vi "登录界面.vi"() -> ()   [LabVIEW 2023]
panel:
  in  "登录":bool
  in  "密   码":string
  in  "用户名":string
  # "登陆界面"
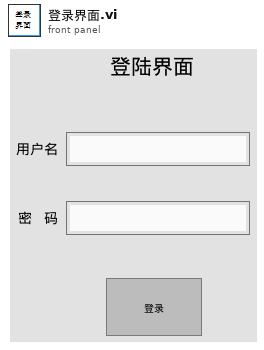
[diagram p1: front panel]
types:
  T1 = enum32{"Invalid", "Standard", "Closed", "Hidden", "Minimized", "Maximized"}
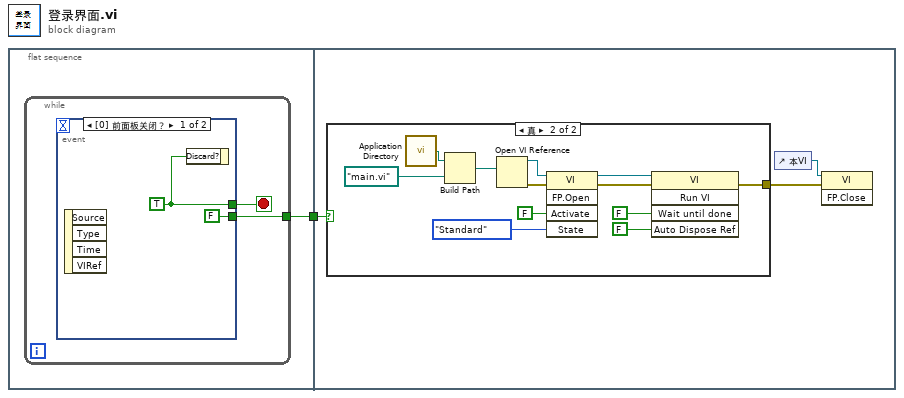
[diagram p0: block diagram]
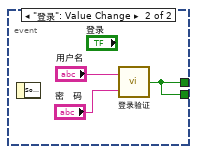
[diagram p2: hidden frame]
diagram:
  n1 = flat-sequence {
    tunnel: [w2] -> w1
    tunnel: w1 -> [w10]
    frame #0 {
      n2 = while {
        tunnel: [w3] -> w2
        stop <- w4 stop-if-true
        n3 = event shown="[0] 前面板关闭？" {
          selector: _ -> [_ _]
          dyn-events: _ -> [_ _]
          timeout: _ -> [_ _]
          tunnel: [w6 w9] -> w4
          tunnel: [FALSE ("是否登录") w9] -> w3
          event Panel Close? {
            w6 = TRUE ("放弃？")
            n4 = event-data() -> ()  [unwired: 1 in, 4 out]
            n5 = event-data("Discard?"=w6) -> ()  [unwired: 1 in, 1 out]
          }
          event "登录": Value Change {
            n6 = event-data() -> ()  [unwired: 1 in, 1 out]
            n7 = call "登录验证.vi"("密   码"="密   码", "用户名"="用户名") -> ("是否登录"=w9:bool)
          }
        }
      }
    }
    frame #1 {
      n8 = case shown="真" w10 {
        tunnel: [_ w15] -> w11
        frame False {
        }
        frame True {
          n9 = call <vilib>:"Application Directory.vi"() -> ("Application Directory"=w24:path)
          n10 = Build Path(base path=w24, name or relative path=path "main.vi" ("名称或相对路径")) -> (appended path=w22:path)
          n11 = Open VI Reference(vi path=w22) -> (vi reference=w21:refnum<vi>, error out=w13:errorcluster)  [unwired: 5 in]
          n12 = invoke class="VI" method="FP.Open"(reference=w21, error in=w13, "Activate"=FALSE ("激活？"), "State"=T1."Standard" ("状态")) -> (reference out=w18:refnum<vi>, error out=w14:errorcluster)  [unwired: 1 in, 3 out]
          n13 = invoke class="VI" method="Run VI"(reference=w18, error in=w14, "Wait until done"=FALSE ("结束前等待"), "Auto Dispose Ref"=FALSE ("自动销毁引用")) -> (error out=w15:errorcluster)  [unwired: 1 in, 4 out]
        }
      }
      n14 = control-ref of="本VI"() -> (w12:refnum<vi>)
      n15 = invoke class="VI" method="FP.Close"(reference=w12, error in=w11) -> ()  [unwired: 1 in, 3 out]
    }
  }
